vi "U8 Performance Test.vi"() -> ()   [LabVIEW 2021]
uses:
  ChannelCommon/typedef/Benchmark Stats.ctl
  ChannelCommon/typedef/Direction.ctl
  ChannelCommon/typedef/FIFO Config.ctl
  CIF_CIPC_Fifo_U8.lvclass
  D:/dev/Packages/CIF_Channels_Core/src/CIFChannels/CIFChannels.lvclass
  ChannelCommon/typedef/New FIFO Instance Configuration.ctl
  <vilib>/Platform/TimedLoop/XDataNode/timing_clust.ctl
  <vilib>/Platform/TimedLoop/XDataNode/nitl_modes.ctl
  <vilib>/Platform/TimedLoop/XDataNode/wakeup.ctl
  ChannelCommon/typedef/TimeStamps.ctl
  CIFChannels/CIFChannels.lvclass/CIFChannels.ctl
  <vilib>/CIF Foundation/CIF Utilities/Statistics/I64/Stats_I64_CIF_U.lvclass/Stats_I64_CIF_U.ctl
  <vilib>/CIF Foundation/CIF Utilities/Statistics/I64/Get Stats.vi
  <vilib>/Platform/TimedLoop/XDataNode/XDataNode.xnode
  <vilib>/Platform/TimedLoop/XDataNode/XDNodeRunTimeDep.lvlib
  ChannelCommon/ChannelCommon.lvlib
  CIFChannels/CIFChannels.lvclass
panel:
  in  "stop":bool
  out "Flatten (us) TO":T1
  out "Channel R/W (us) TO":T1
  out "Flatten (us)":T1
  out "Channel R/W (us)":T1
  out "avg TO":dbl
  out "max TO":dbl
  out "timed out? 3":bool
  out "timed out?":bool
  out "avg channel":dbl
  out "max channel":dbl
  out "pass":bool
  out "error out":errorcluster
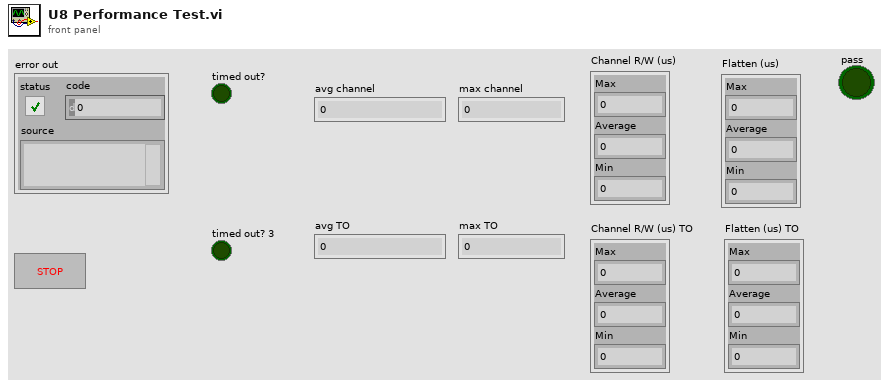
[diagram p1: front panel]
types:
  T1 = typedef "ChannelCommon.lvlib/Benchmark Stats.ctl" = cluster{"Max":i64, "Average":dbl, "Min":i64}
  T2 = typedef "ChannelCommon.lvlib/FIFO Config.ctl" = cluster{"Max Bytes/Msg":u64, "Max Msg/FIFO":u64, "Flags":u64, "Custom Data":u8[]}
  T3 = typedef "ChannelCommon.lvlib/Direction.ctl" = enum8{"Publisher", "Subscriber"}
  T4 = typedef "ChannelCommon.lvlib/New FIFO Instance Configuration.ctl" = cluster{"Backpressure":bool, "Bytes/Message Override":u32, "Messages/FIFO Override":u32, "Custom Data":u8[]}
  T5 = typedef "ChannelCommon.lvlib/TimeStamps.ctl" = cluster{"ClockID":u8, "T0":i64, "T_Out":i64}
  T6 = typedef "XDNodeRunTimeDep.lvlib/timing_clust.ctl" = cluster{"Expected End [f-1]":u64, "Actual End [f-1]":u64, "Finished Late? [f-1]":bool, "Expected End [i-1]":u64, "Actual End [i-1]":u64, "Finished Late? [i-1]":bool, "Expected Start [i]":u64, "Actual Start [i]":u64, "Expected Start [f]":u64, "Actual Start [f]":u64, "Source Name":string, "Structure Name":string, "Period":i64, "Deadline":i64, "Offset":i64, "Start":i64, "Priority":i32, "Timeout":i32, "Mode":T7, "Wakeup Reason":T8, "Error":errorcluster, "Source Type":string, "Secondary Source Type":string, "Global End Time":u64, "Global Start Time":u64, "Frame Duration":u64, "Iteration Duration":u64, "Assigned CPU":i32, "I/O Scan Engine Mode":u32}
  T7 = typedef "XDNodeRunTimeDep.lvlib/nitl_modes.ctl" = enum32{"No Change", "Process missed periods, maintain original phase", "Discard missed periods, maintain original phase", "Process missed periods, ignore original phase", "Discard missed periods, ignore original phase"}
  T8 = typedef "XDNodeRunTimeDep.lvlib/wakeup.ctl" = enum32{"Normal", "Aborted", "Asynchronous wakeup", "Timing source error", "Timed loop error", "Timeout"}
  T9 = typedef "ChannelCommon.lvlib/New FIFO Instance Response.ctl" = cluster{"Publisher":string, "Custom Data":u8[]}
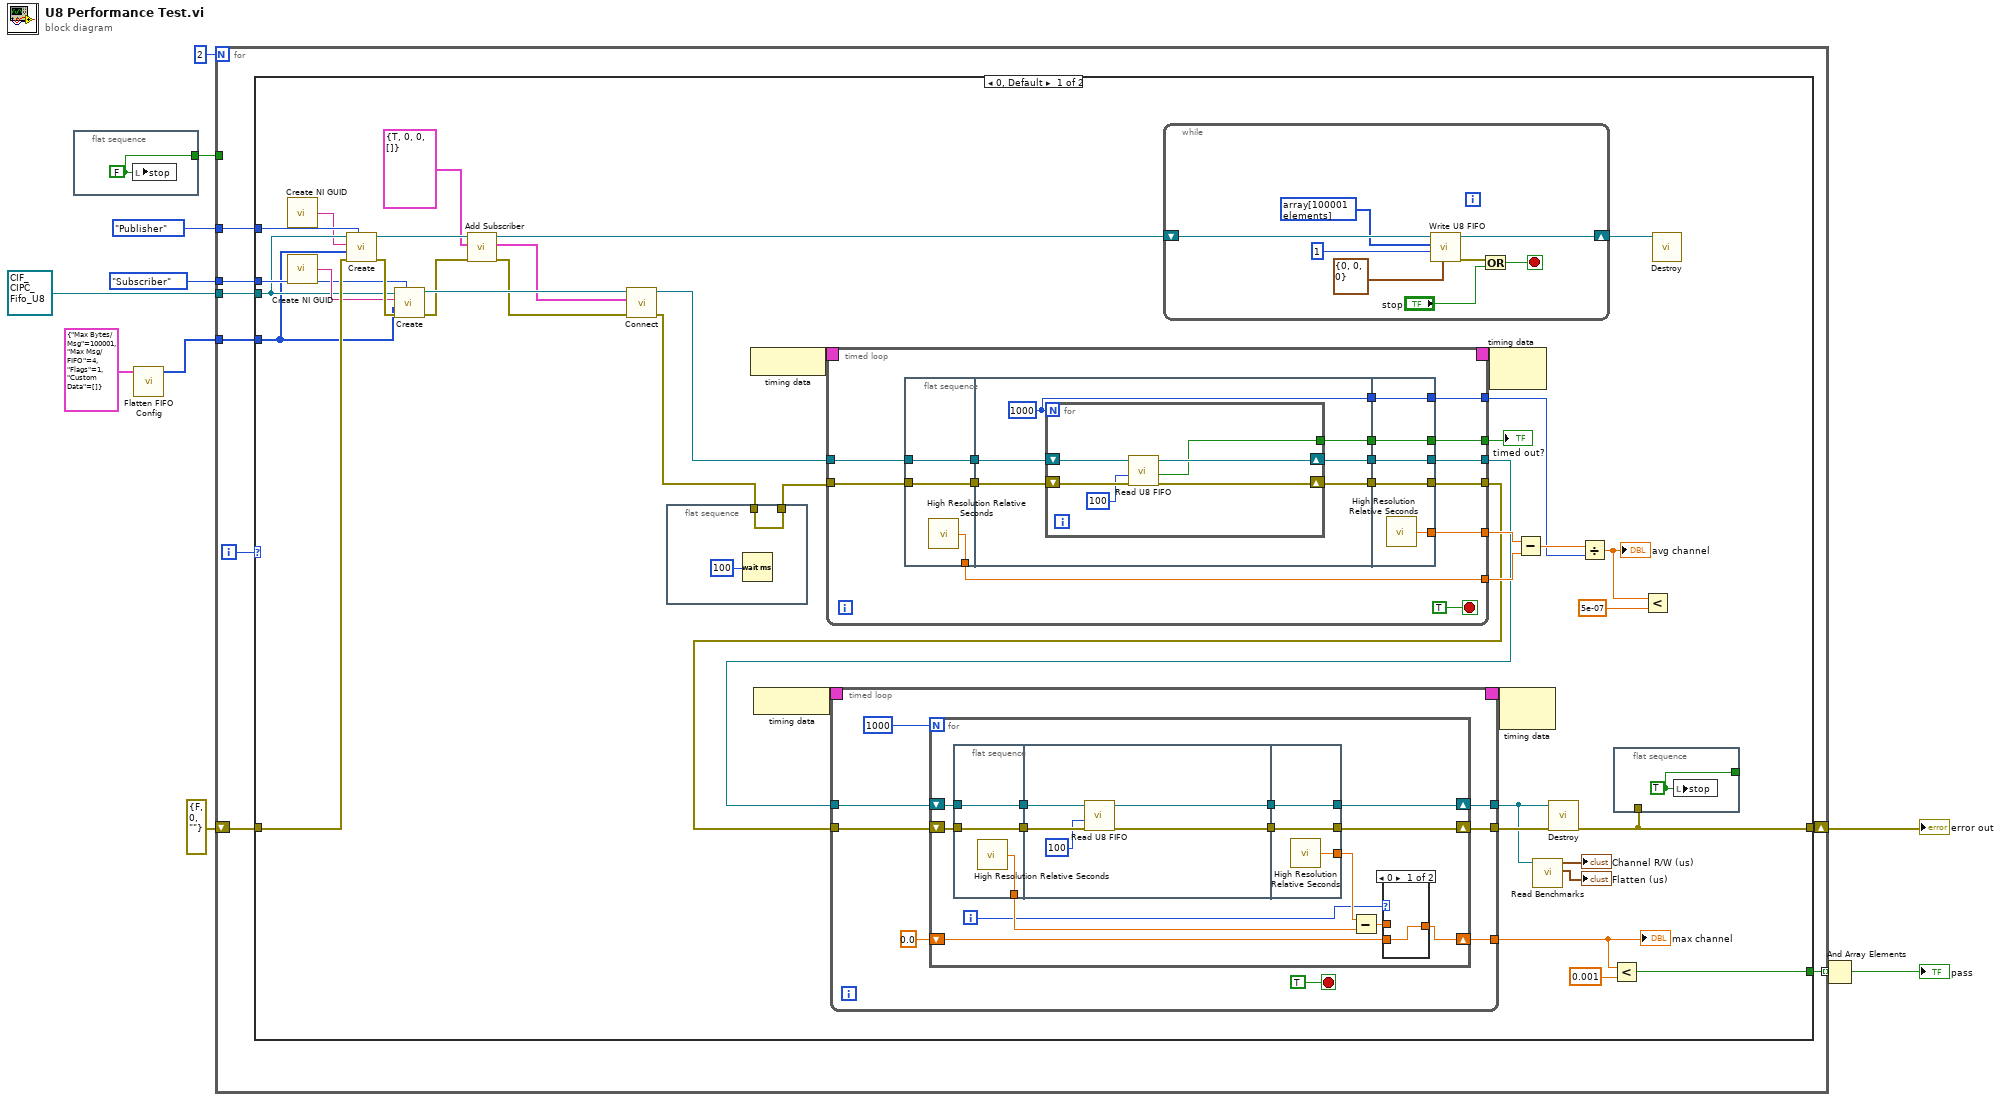
[diagram p0: block diagram]
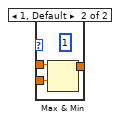
[diagram p2: hidden frame]
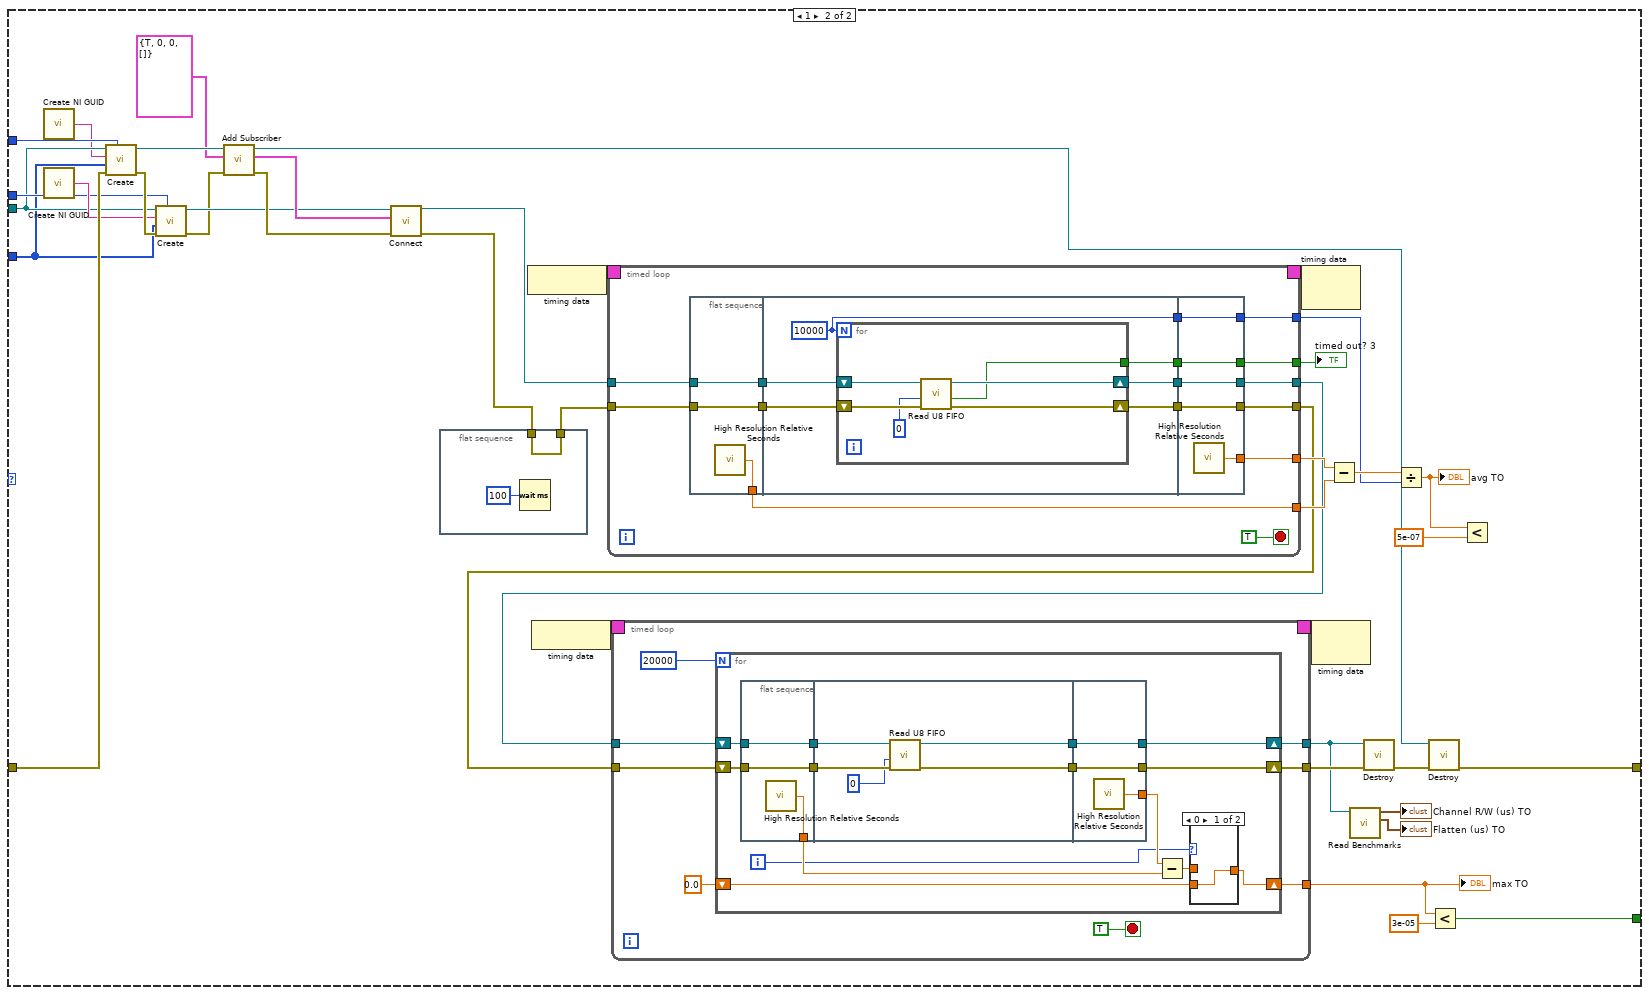
[diagram p3: hidden frame]
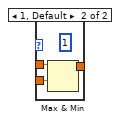
[diagram p4: hidden frame]
diagram:
  n1 = flat-sequence {
    tunnel: [w12] -> w1
    frame #0 {
      w12 = FALSE ("stop")
      n2 = local write "stop"(w12) -> ()
    }
  }
  n3 = call "Flatten FIFO Config.vi"("FIFO Config in"=T2 {"Max Bytes/Msg"=100001, "Max Msg/FIFO"=4, "Flags"=1, "Custom Data"=[]}) -> ("Flattened FIFO Config"=w3:u8[])  [unwired: 10 in]
  n4 = for {
    N: 2 -> [_]
    tunnel: [w20] -> w9 mode=indexing
    shift-right: [w19] -> w11
    shift-left: errorcluster {"status"=FALSE, "code"=0, "source"=""} ("error out") -> [w17]
    tunnel: Direction."Publisher" ("Direction") -> [w16]
    tunnel: Direction."Subscriber" ("Direction") -> [w15]
    tunnel: refnum<class "CIF_CIPC_Fifo_U8.lvclass"> refnum ("CIF_CIPC_Fifo_U8.lvclass") -> [w14]
    tunnel: w3 -> [w13]
    tunnel: w1 -> [_]
    i -> [w18]
    n5 = case shown="0, Default" w18 {
      tunnel: [w46 w177] -> w20
      tunnel: [w27 w166] -> w19
      tunnel: w17 -> [w44 w175]
      tunnel: w16 -> [w42 w173]
      tunnel: w15 -> [w41 w172]
      tunnel: w14 -> [w40 w171]
      tunnel: w13 -> [w37 w169]
      frame 0, Default {
        n6 = call <vilib>:"Create NI GUID.vi"() -> ("NI GUID"=w38:string)
        n7 = call <vilib>:"Create NI GUID.vi"() -> ("NI GUID"=w43:string)
        n8 = call-dynamic "Create.vi"("Direction"=w42, "error in (no error)"=w44, "Custom Config Data"=w37, "Name"=w38, "CIFFIFO in"=w40) -> ("error out"=w45:errorcluster, "CIFFIFO out"=w26:refnum<class "CIF_CIPC_Fifo_U8.lvclass">)  [unwired: 5 in]
        n9 = call-dynamic "Create.vi"("Direction"=w41, "error in (no error)"=w45, "Custom Config Data"=w37, "Name"=w43, "CIFFIFO in"=w40) -> ("error out"=w24:errorcluster, "CIFFIFO out"=w39:refnum<class "CIF_CIPC_Fifo_U8.lvclass">)  [unwired: 5 in]
        n10 = call-dynamic "Add Subscriber.vi"("error in (no error)"=w24, "New FIFO Instance Config"=T4 {"Backpressure"=TRUE, "Bytes/Message Override"=0, "Messages/FIFO Override"=0, "Custom Data"=[]}, "CIF_CIPC_Chn in"=w26) -> ("error out"=w23:errorcluster, "New FIFO Instance"=w22:T9, "CIF_CIPC_Chn out"=w25:refnum<class "CIF_CIPC_Fifo_U8.lvclass">)  [unwired: 6 in]
        n11 = call-dynamic "Connect.vi"("error in (no error)"=w23, "Connection"=w22, "CIFTag in"=w39) -> ("error out"=w34:errorcluster, "CIFTag out"=w36:refnum<class "CIF_CIPC_Fifo_U8.lvclass">)  [unwired: 7 in]
        n12 = flat-sequence {
          tunnel: w34 -> [w63]
          tunnel: [w63] -> w33
          frame #0 {
            n13 = Wait (ms)(milliseconds to wait=u32 100) -> ()  [unwired: 1 out]
          }
        }
        n14 = node-c288() -> (w60:T6)
        n15 = node-c288() -> (w58:T6)
        n16 = timed-loop {
          timing: w60 -> [_]
          timing-out: [_] -> w59
          tunnel: w36 -> [w127]
          tunnel: w33 -> [w126]
          tunnel: [w122] -> w52
          tunnel: [w120] -> w51
          tunnel: [w118] -> w56
          tunnel: [w117] -> w55
          tunnel: [w116] -> w53
          tunnel: [w114] -> w32
          stop <- TRUE stop-if-true
          n17 = flat-sequence {
            tunnel: w126 -> [w129]
            tunnel: w127 -> [w130]
            tunnel: [w130] -> w124
            tunnel: [w129] -> w123
            tunnel: [w128] -> w117
            tunnel: w124 -> [w136]
            tunnel: w123 -> [w135]
            tunnel: [w134] -> w121
            tunnel: [w133] -> w119
            tunnel: [w132] -> w115
            tunnel: [w131] -> w113
            tunnel: [w147] -> w122
            tunnel: w121 -> [w147]
            tunnel: [w146] -> w120
            tunnel: w119 -> [w146]
            tunnel: [w145] -> w118
            tunnel: [w144] -> w116
            tunnel: w115 -> [w144]
            tunnel: [w143] -> w114
            tunnel: w113 -> [w143]
            frame #0 {
              n18 = call <vilib>:"High Resolution Relative Seconds.vi"() -> ("relative seconds"=w128:dbl)
            }
            frame #1 {
              w132 = 1000
              n19 = for {
                N: w132 -> [_]
                shift-right: [w139] -> w134
                shift-left: w136 -> [w142]
                shift-right: [w140] -> w133
                shift-left: w135 -> [w141]
                tunnel: [w137] -> w131
                n20 = call-dynamic "Read U8 FIFO.vi"("error in (no error)"=w141, "Timeout (ms)"=100, "CIFFIFO in"=w142) -> ("error out"=w140:errorcluster, "timed out?"=w137:bool, "CIFFIFO out"=w139:refnum<class "CIF_CIPC_Fifo_U8.lvclass">)  [unwired: 4 in, 2 out]
              }
            }
            frame #2 {
              n21 = call <vilib>:"High Resolution Relative Seconds.vi"() -> ("relative seconds"=w145:dbl)
            }
          }
        }
        "timed out?" <- w32
        n22 = timed-loop {
          timing: w58 -> [_]
          timing-out: [_] -> w57
          tunnel: w52 -> [w79]
          tunnel: w51 -> [w78]
          tunnel: [w76] -> w31
          tunnel: [w75] -> w35
          tunnel: [w72] -> w48
          stop <- TRUE stop-if-true
          n23 = for {
            N: 1000 -> [_]
            shift-right: [w88] -> w76
            shift-left: w79 -> [w90]
            shift-right: [w87] -> w75
            shift-left: w78 -> [w89]
            shift-right: [w82] -> w72
            shift-left: 0.0 -> [w83]
            i -> [w81]
            n24 = flat-sequence {
              tunnel: w89 -> [w99]
              tunnel: w90 -> [w100]
              tunnel: [w100] -> w93
              tunnel: [w99] -> w92
              tunnel: [w98] -> w85
              tunnel: w93 -> [w105]
              tunnel: w92 -> [w104]
              tunnel: [w102] -> w91
              tunnel: [w103] -> w80
              tunnel: [w108] -> w88
              tunnel: w91 -> [w108]
              tunnel: [w107] -> w87
              tunnel: [w106] -> w86
              tunnel: w80 -> [w107]
              frame #0 {
                n25 = call <vilib>:"High Resolution Relative Seconds.vi"() -> ("relative seconds"=w98:dbl)
              }
              frame #1 {
                n26 = call-dynamic "Read U8 FIFO.vi"("error in (no error)"=w104, "Timeout (ms)"=100, "CIFFIFO in"=w105) -> ("error out"=w103:errorcluster, "CIFFIFO out"=w102:refnum<class "CIF_CIPC_Fifo_U8.lvclass">)  [unwired: 4 in, 3 out]
              }
              frame #2 {
                n27 = call <vilib>:"High Resolution Relative Seconds.vi"() -> ("relative seconds"=w106:dbl)
              }
            }
            n28 = Subtract(x=w86, y=w85) -> (x-y=w84:dbl)
            n29 = case shown="0" w81 {
              tunnel: w84 -> [_ w97]
              tunnel: w83 -> [w94 w96]
              tunnel: [w94 w95] -> w82
              frame 0 {
              }
              frame 1, Default {
                (unwired) u32 1 ("milliseconds to wait")
                n30 = Max & Min(x=w97, y=w96) -> (max(x,y)=w95:dbl)  [unwired: 1 out]
              }
            }
          }
        }
        "max channel" <- w48
        n31 = while {
          shift-right: [w69] -> w28
          shift-left: w25 -> [w71]
          stop <- w66 stop-if-true
          n32 = call-dynamic "Write U8 FIFO.vi"("FIFO Timestamps"=T5 {"ClockID"=0, "T0"=0, "T_Out"=0}, "Timeout (ms)"=1, "Data in"=u8[] array[100001 elements] ("U8 Data"), "CIFFIFO in"=w71) -> ("error out"=w67:errorcluster, "CIFFIFO out"=w69:refnum<class "CIF_CIPC_Fifo_U8.lvclass">)  [unwired: 4 in, 2 out]
          n33 = Or(x=w67, y="stop") -> (x .or. y?=w66:bool)
        }
        n34 = node-c288(w59) -> ()  [unwired: 1 out]
        n35 = node-c288(w57) -> ()  [unwired: 1 out]
        n36 = Subtract(x=w56, y=w55) -> (x-y=w54:dbl)
        n37 = call "Read Benchmarks.vi"("CIFChannels in"=w31) -> ("Flatten (us)"=→"Flatten (us)":T1, "Channel R/W (us)"=→"Channel R/W (us)":T1)  [unwired: 9 in]
        n38 = call-dynamic "Destroy.vi"("error in (no error)"=w35, "CIFTag in"=w31) -> ("error out"=w27:errorcluster)  [unwired: 8 in, 1 out]
        n39 = Divide(x=w54, y=w53) -> (x/y=w50:dbl)
        "avg channel" <- w50
        n40 = Less?(x=w48, y=0.001) -> (x < y?=w46:bool)
        n41 = flat-sequence {
          tunnel: [w61] -> _
          tunnel: w27 -> [_]
          frame #0 {
            w61 = TRUE ("stop")
            n42 = local write "stop"(w61) -> ()
          }
        }
        n43 = Less?(x=w50, y=5e-07) -> ()  [unwired: 1 out]
        n44 = call-dynamic "Destroy.vi"("CIFTag in"=w28) -> ()  [unwired: 9 in, 2 out]
      }
      frame 1 {
        n45 = call <vilib>:"Create NI GUID.vi"() -> ("NI GUID"=w170:string)
        n46 = call <vilib>:"Create NI GUID.vi"() -> ("NI GUID"=w174:string)
        n47 = call-dynamic "Create.vi"("Direction"=w173, "error in (no error)"=w175, "Custom Config Data"=w169, "Name"=w170, "CIFFIFO in"=w171) -> ("error out"=w176:errorcluster, "CIFFIFO out"=w157:refnum<class "CIF_CIPC_Fifo_U8.lvclass">)  [unwired: 5 in]
        n48 = call-dynamic "Create.vi"("Direction"=w172, "error in (no error)"=w176, "Custom Config Data"=w169, "Name"=w174, "CIFFIFO in"=w171) -> ("error out"=w156:errorcluster, "CIFFIFO out"=w158:refnum<class "CIF_CIPC_Fifo_U8.lvclass">)  [unwired: 5 in]
        n49 = call-dynamic "Add Subscriber.vi"("error in (no error)"=w156, "New FIFO Instance Config"=T4 {"Backpressure"=TRUE, "Bytes/Message Override"=0, "Messages/FIFO Override"=0, "Custom Data"=[]}, "CIF_CIPC_Chn in"=w157) -> ("error out"=w160:errorcluster, "New FIFO Instance"=w159:T9, "CIF_CIPC_Chn out"=w153:refnum<class "CIF_CIPC_Fifo_U8.lvclass">)  [unwired: 6 in]
        n50 = call-dynamic "Connect.vi"("error in (no error)"=w160, "Connection"=w159, "CIFTag in"=w158) -> ("error out"=w155:errorcluster, "CIFTag out"=w154:refnum<class "CIF_CIPC_Fifo_U8.lvclass">)  [unwired: 7 in]
        n51 = flat-sequence {
          tunnel: w155 -> [w193]
          tunnel: [w193] -> w165
          frame #0 {
            n52 = Wait (ms)(milliseconds to wait=u32 100) -> ()  [unwired: 1 out]
          }
        }
        n53 = node-c288() -> (w191:T6)
        n54 = node-c288() -> (w189:T6)
        n55 = timed-loop {
          timing: w191 -> [_]
          timing-out: [_] -> w190
          tunnel: w154 -> [w249]
          tunnel: w165 -> [w248]
          tunnel: [w244] -> w183
          tunnel: [w242] -> w182
          tunnel: [w240] -> w187
          tunnel: [w239] -> w186
          tunnel: [w238] -> w184
          tunnel: [w236] -> w164
          stop <- TRUE stop-if-true
          n56 = flat-sequence {
            tunnel: w248 -> [w251]
            tunnel: w249 -> [w252]
            tunnel: [w252] -> w246
            tunnel: [w251] -> w245
            tunnel: [w250] -> w239
            tunnel: w246 -> [w258]
            tunnel: w245 -> [w257]
            tunnel: [w256] -> w243
            tunnel: [w255] -> w241
            tunnel: [w254] -> w237
            tunnel: [w253] -> w235
            tunnel: [w269] -> w244
            tunnel: w243 -> [w269]
            tunnel: [w268] -> w242
            tunnel: w241 -> [w268]
            tunnel: [w267] -> w240
            tunnel: [w266] -> w238
            tunnel: w237 -> [w266]
            tunnel: [w265] -> w236
            tunnel: w235 -> [w265]
            frame #0 {
              n57 = call <vilib>:"High Resolution Relative Seconds.vi"() -> ("relative seconds"=w250:dbl)
            }
            frame #1 {
              w254 = 10000
              n58 = for {
                N: w254 -> [_]
                shift-right: [w261] -> w256
                shift-left: w258 -> [w264]
                shift-right: [w262] -> w255
                shift-left: w257 -> [w263]
                tunnel: [w260] -> w253
                n59 = call-dynamic "Read U8 FIFO.vi"("error in (no error)"=w263, "Timeout (ms)"=0, "CIFFIFO in"=w264) -> ("error out"=w262:errorcluster, "timed out?"=w260:bool, "CIFFIFO out"=w261:refnum<class "CIF_CIPC_Fifo_U8.lvclass">)  [unwired: 4 in, 2 out]
              }
            }
            frame #2 {
              n60 = call <vilib>:"High Resolution Relative Seconds.vi"() -> ("relative seconds"=w267:dbl)
            }
          }
        }
        "timed out? 3" <- w164
        n61 = timed-loop {
          timing: w189 -> [_]
          timing-out: [_] -> w188
          tunnel: w183 -> [w201]
          tunnel: w182 -> [w200]
          tunnel: [w198] -> w161
          tunnel: [w197] -> w168
          tunnel: [w194] -> w179
          stop <- TRUE stop-if-true
          n62 = for {
            N: 20000 -> [_]
            shift-right: [w210] -> w198
            shift-left: w201 -> [w212]
            shift-right: [w209] -> w197
            shift-left: w200 -> [w211]
            shift-right: [w204] -> w194
            shift-left: 0.0 -> [w205]
            i -> [w203]
            n63 = flat-sequence {
              tunnel: w211 -> [w221]
              tunnel: w212 -> [w222]
              tunnel: [w222] -> w215
              tunnel: [w221] -> w214
              tunnel: [w220] -> w207
              tunnel: w215 -> [w227]
              tunnel: w214 -> [w225]
              tunnel: [w226] -> w213
              tunnel: [w224] -> w202
              tunnel: [w230] -> w210
              tunnel: w213 -> [w230]
              tunnel: [w229] -> w209
              tunnel: [w228] -> w208
              tunnel: w202 -> [w229]
              frame #0 {
                n64 = call <vilib>:"High Resolution Relative Seconds.vi"() -> ("relative seconds"=w220:dbl)
              }
              frame #1 {
                n65 = call-dynamic "Read U8 FIFO.vi"("error in (no error)"=w225, "Timeout (ms)"=0, "CIFFIFO in"=w227) -> ("error out"=w224:errorcluster, "CIFFIFO out"=w226:refnum<class "CIF_CIPC_Fifo_U8.lvclass">)  [unwired: 4 in, 3 out]
              }
              frame #2 {
                n66 = call <vilib>:"High Resolution Relative Seconds.vi"() -> ("relative seconds"=w228:dbl)
              }
            }
            n67 = Subtract(x=w208, y=w207) -> (x-y=w206:dbl)
            n68 = case shown="0" w203 {
              tunnel: w206 -> [_ w219]
              tunnel: w205 -> [w216 w218]
              tunnel: [w216 w217] -> w204
              frame 0 {
              }
              frame 1, Default {
                (unwired) u32 1 ("milliseconds to wait")
                n69 = Max & Min(x=w219, y=w218) -> (max(x,y)=w217:dbl)  [unwired: 1 out]
              }
            }
          }
        }
        "max TO" <- w179
        n70 = node-c288(w190) -> ()  [unwired: 1 out]
        n71 = node-c288(w188) -> ()  [unwired: 1 out]
        n72 = Subtract(x=w187, y=w186) -> (x-y=w185:dbl)
        n73 = call "Read Benchmarks.vi"("CIFChannels in"=w161) -> ("Flatten (us)"=→"Flatten (us) TO":T1, "Channel R/W (us)"=→"Channel R/W (us) TO":T1)  [unwired: 9 in]
        n74 = call-dynamic "Destroy.vi"("error in (no error)"=w168, "CIFTag in"=w161) -> ("error out"=w167:errorcluster)  [unwired: 8 in, 1 out]
        n75 = Divide(x=w185, y=w184) -> (x/y=w181:dbl)
        "avg TO" <- w181
        n76 = call-dynamic "Destroy.vi"("error in (no error)"=w167, "CIFTag in"=w153) -> ("error out"=w166:errorcluster)  [unwired: 8 in, 1 out]
        n77 = Less?(x=w179, y=3e-05) -> (x < y?=w177:bool)
        n78 = Less?(x=w181, y=5e-07) -> ()  [unwired: 1 out]
      }
    }
  }
  "error out" <- w11
  n79 = And Array Elements(Boolean array=w9) -> (logical AND=→"pass":bool)
